vi "DetectedPeaksToTDMS.vi"(11 "Detected peaks":T1[](array[typedef])) -> (3 "Array":dbl[][](array[numeric]))   [LabVIEW 2021]
uses:
  Typedefs/Detected peaks.ctl
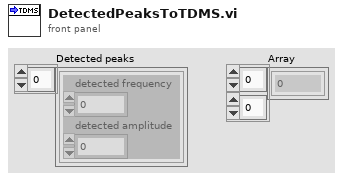
[diagram p1: front panel]
types:
  T1 = typedef "Detected peaks.ctl" = cluster{"detected frequency":dbl, "detected amplitude":dbl}
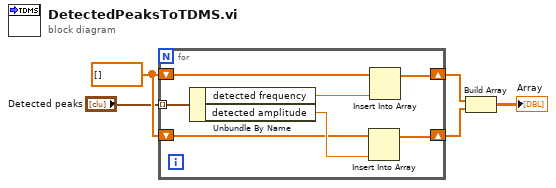
[diagram p0: block diagram]
diagram:
  w2 = dbl[] []
  n1 = for {
    tunnel: "Detected peaks" -> [w12] mode=indexing
    shift-right: [w10] -> w3
    shift-left: w2 -> [w9]
    shift-right: [w7] -> w4
    shift-left: w2 -> [w6]
    n2 = Unbundle By Name(w12) -> ("detected frequency"=w11:dbl, "detected amplitude"=w8:dbl)
    n3 = Insert Into Array(array=w6, new element=w8) -> (w7:dbl[])  [unwired: 1 in]
    n4 = Insert Into Array(array=w9, new element=w11) -> (w10:dbl[])  [unwired: 1 in]
  }
  n5 = Build Array(w3, w4) -> (→"Array":dbl[][])
